vi "Get Instances Helper.vi"   [LabVIEW 2019, in "Lookup API.lvlib"]
doc: "<b>Description</b> A helper VI snippet for use with the Lookup API. Drop the contents of this VI directly onto your block diagram.\n\nAfter dropping this in your VI, follow the instructions in the labels to update the types."
uses:
  Lookup API.lvlib
  ede7ea97-040b-4829-825c-5958a8520bea.vi
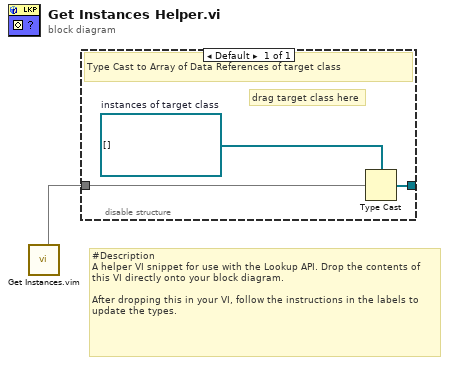
[diagram p0: block diagram]
diagram:
  # "#Description\nA helper VI snippet for use with the Lookup API. Drop the contents of this VI directly onto your block diagram.\n\nAfter dropping this in your VI, follow the instructions in the labels to update the types."
  n1 = call "Get Instances.vim"() -> ("instances"=w1:set{refnum<data-value>})  [unwired: 9 in, 2 out]
  n2 = disable-structure shown="Default" {
    disable-tunnel: w1 -> [w4]
    disable-tunnel: [w2] -> _
    frame Enabled {
      w3 = refnum<data-value>[] []  # instances of target class
      # "drag target class here"
      # "Type Cast to Array of Data References of target class"
      n3 = Type Cast(type=w3, x=w4) -> (*(type *) &x=w2:refnum<data-value>[])
    }
  }
